vi "usrp TX.vi"() -> ()   [LabVIEW 2019]
uses:
  <instrlib>/niUSRP/niUSRP Write Tx Data (CDB Cluster).vi
  <vilib>/addons/Modulation/Digital/General/MT Generate PSK System Parameters(M).vi
  <vilib>/addons/Modulation/niDMT.lvlib
panel:
  in  "Modulation type":string(combo)="QPSK"
  in  "16-PSK System Parameters 2":T1={"Samples per Symbol"=8, "symbol map"=[], "Differential PSK"=enum."disable", "PSK type"=0} caption="16-PSK System Parameters" {"PSK type" items=["normal", "shifted", "offset"]; "symbol map" format="%.3f"}
  in  "8-PSK System Parameters 2":T1={"Samples per Symbol"=8, "symbol map"=[], "Differential PSK"=enum."disable", "PSK type"=0} caption="8-PSK System Parameters" {"PSK type" items=["normal", "shifted", "offset"]; "symbol map" format="%.3f"}
  in  "QPSK System Parameters 2":T1={"Samples per Symbol"=8, "symbol map"=[], "Differential PSK"=enum."disable", "PSK type"=0} caption="QPSK System Parameters" {"PSK type" items=["normal", "shifted", "offset"]; "symbol map" format="%.3f"}
  in  "BPSK System Parameters 2":T1={"Samples per Symbol"=8, "symbol map"=[], "Differential PSK"=enum."disable", "PSK type"=0} caption="BPSK System Parameters" {"PSK type" items=["normal", "shifted", "offset"]; "symbol map" format="%.3f"}
  in  "PN sequence order\nfor Sync Bits":i32=31 caption="PN sequence order (9)"
  in  "USRP IP address":refnum<k15>="192.168.10.2"
  in  "Packet Pad \n[samples]":i32=200
  out "Number of Packets in Message":i32=46
  in  "Message Text":string="Two roads diverged in a yellow wood,\nAnd sorry I could not travel both\nAnd be one traveler, long I stood\nAnd looked down one as far as I could\nTo where it bent in the undergrowth.\n\nThen took the other, as just as fair,\nAnd having perhaps the better claim,\nBecause it was grassy and wanted wear;\nThough as for that the passing there\nHad worn them really about the same.\n\nAnd both that morning equally lay\nIn leaves no step had trodden black.\nOh, I kept the first for another day!\nYet knowing how way leads on to way,\nI doubted if I should ever come back.\n\nI shall be telling this with a sigh\nSomewhere ages and ages hence:\nTwo roads diverged in a wood, and I--\nI took the one less traveled by,\nAnd that has made all the difference.\n"
  in  "Message Type":bool=TRUE
  in  "Tx Parameters":T2={"Tx IQ Sampling\nRate [s/sec]"=400000.0, "Tx Frequency [Hz]"=915000000.0, "Tx Gain [dB]"=0.0, "Tx Antenna"="TX1"} {"Tx Gain [dB]" format="%#.6p"; "Tx Frequency [Hz]" format="%#.6p"; "Tx IQ Sampling\nRate [s/sec]" format="%#.6p"}
  out "Actual Tx Parameters":T2={"Tx IQ Sampling\nRate [s/sec]"=400000.0, "Tx Frequency [Hz]"=915000000.0, "Tx Gain [dB]"=0.0, "Tx Antenna"="TX1"} {"Tx Gain [dB]" format="%#.6p"; "Tx Frequency [Hz]" format="%#.6p"; "Tx IQ Sampling\nRate [s/sec]" format="%#.6p"}
  in  "Packet Parameters":T3={"Guard Bits "=30, "Sync Bits"=20, "Message Bits"=128}
  out "error out":errorcluster
  out "Constellation Graph":T4(graph)
  in  "autoscale":bool
  out "Transmitted Signal":cluster{"t0":dbl, "dt":dbl, "Y":dbl[]}(graph)
  in  "Queue Length":i32=10
  in  "Blank Frame \n[samples]":i32=500
  in  "Pulse Shaping Filter Parameters":T5={"Alpha"=0.5, "Filter Length"=6, "TX Filter"=enum."Root Raised Cos"} caption="Pulse Shaping Filter" {"Alpha" format="%.2f"}
  out "Symbol Rate [symbols/sec]":dbl=50000.0 format="%#.6p"
  in  "stop":bool
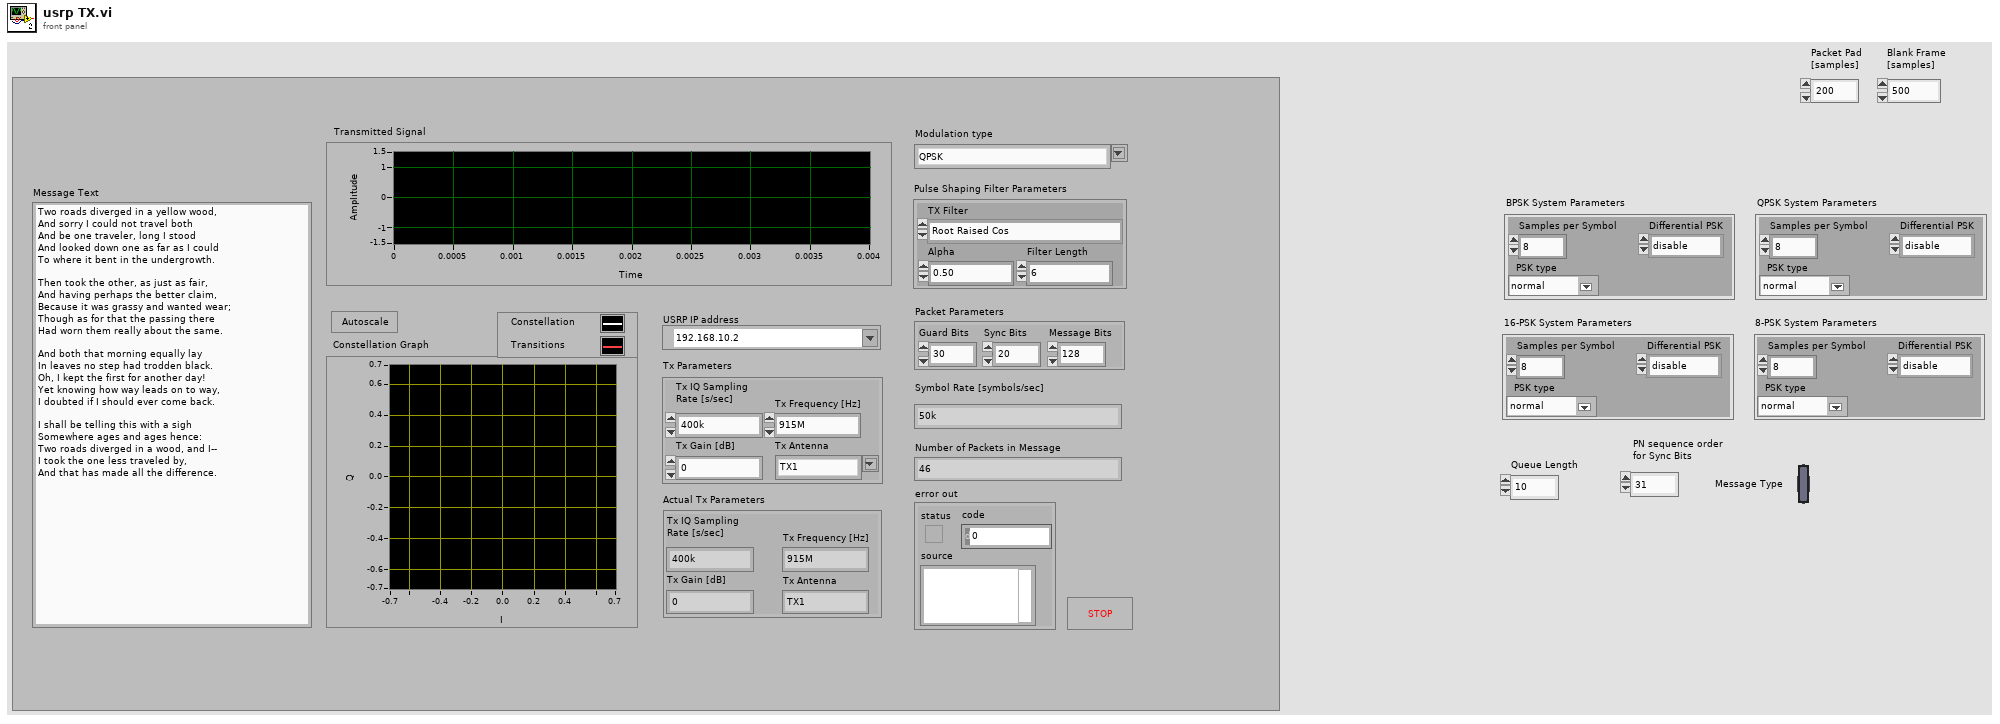
[diagram p1: front panel]
types:
  T1 = cluster{"Samples per Symbol":i32, "symbol map":cdb[], "Differential PSK":enum16{"disable", "enable"}, "PSK type":u16}
  T2 = cluster{"Tx IQ Sampling\nRate [s/sec]":dbl, "Tx Frequency [Hz]":dbl, "Tx Gain [dB]":dbl, "Tx Antenna":string}
  T3 = cluster{"Guard Bits ":i32, "Sync Bits":i32, "Message Bits":i32}
  T4 = cluster{"Decimated Array":dbl[], "Decimated Array":dbl[]}[]
  T5 = cluster{"Alpha":dbl, "Filter Length":i32, "TX Filter":enum16{"none", "Raised Cosine", "Root Raised Cos", "Gaussian"}}
  T6 = cluster{"samples per symbol (16)":i32, "symbol map":cdb[], "differential PSK":enum16{"disable", "enable"}, "PSK type":u16}
  T7 = cluster{"s? t:f":cluster{"t0":dbl, "dt":dbl, "Y":cdb[]}, i32}
  T8 = cluster{"output complex waveform":cluster{"t0":dbl, "dt":dbl, "Y":cdb[]}, i32}
  T9 = cluster{"constellation":dbl[], "oversampled data":dbl[]}[]
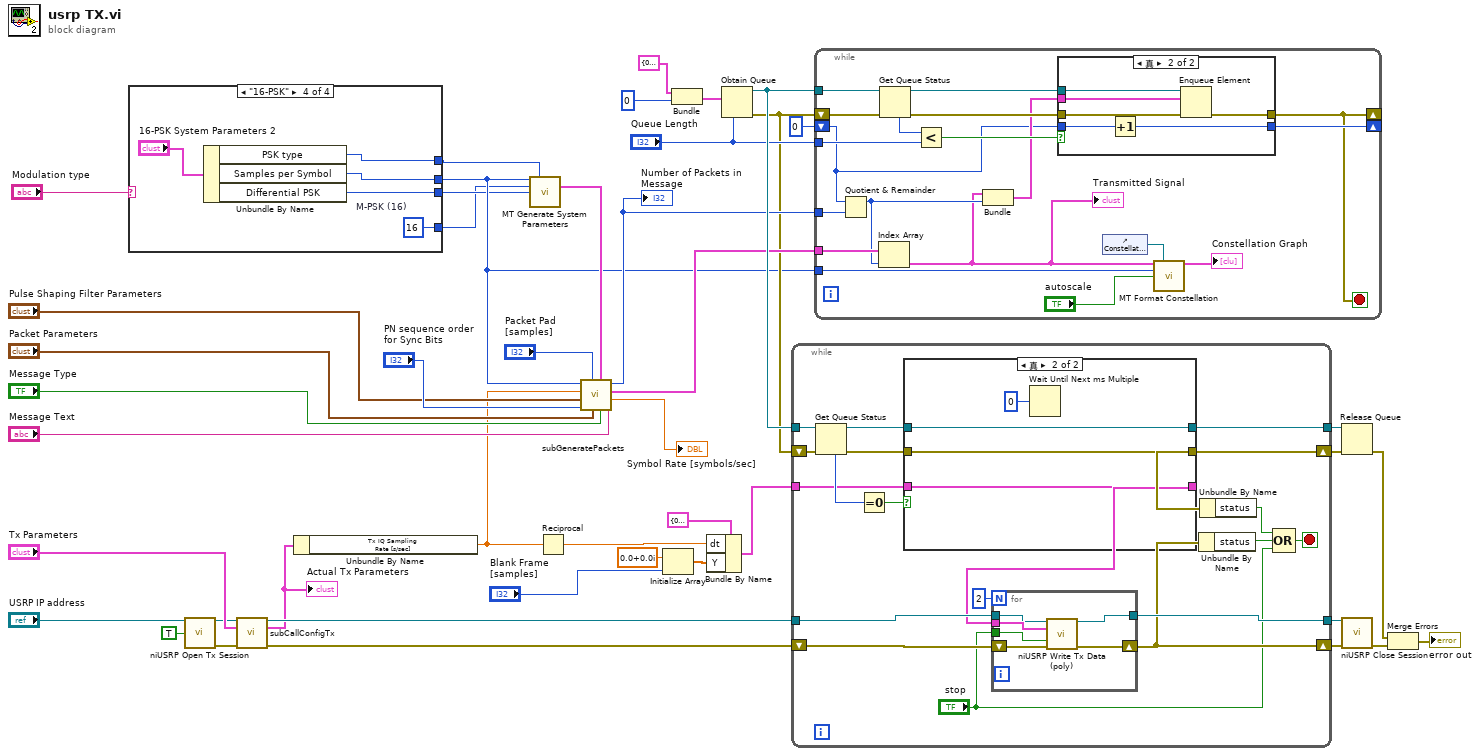
[diagram p0: block diagram]
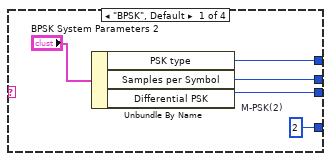
[diagram p2: hidden frame]
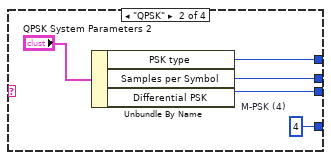
[diagram p3: hidden frame]
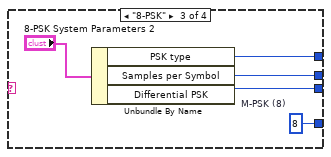
[diagram p4: hidden frame]
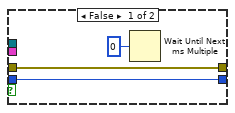
[diagram p5: hidden frame]
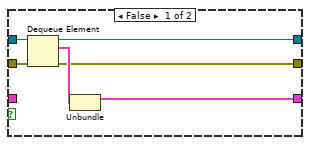
[diagram p6: hidden frame]
diagram:
  n1 = case shown="\"16-PSK\"" "Modulation type" {
    tunnel: [w46 w50 w58 w64] -> w3
    tunnel: [w47 w52 w57 w63] -> w2
    tunnel: [w49 w54 w56 w62] -> w1
    tunnel: [w48 w53 w59 w61] -> w4
    frame "BPSK", Default {
      w49 = 2  # M-PSK(2)
      n2 = Unbundle By Name("BPSK System Parameters 2") -> ("PSK type"=w48:u16, "Samples per Symbol"=w46:i32, "Differential PSK"=w47:enum16{"disable", "enable"})
    }
    frame "QPSK" {
      w54 = 4  # M-PSK (4)
      n3 = Unbundle By Name("QPSK System Parameters 2") -> ("PSK type"=w53:u16, "Samples per Symbol"=w50:i32, "Differential PSK"=w52:enum16{"disable", "enable"})
    }
    frame "8-PSK" {
      w56 = 8  # M-PSK (8)
      n4 = Unbundle By Name("8-PSK System Parameters 2") -> ("PSK type"=w59:u16, "Samples per Symbol"=w58:i32, "Differential PSK"=w57:enum16{"disable", "enable"})
    }
    frame "16-PSK" {
      w62 = 16  # M-PSK (16)
      n5 = Unbundle By Name("16-PSK System Parameters 2") -> ("PSK type"=w61:u16, "Samples per Symbol"=w64:i32, "Differential PSK"=w63:enum16{"disable", "enable"})
    }
  }
  n6 = call <instrlib>:"niUSRP Open Tx Session.vi"("device names"="USRP IP address", "reset"=TRUE) -> ("session handle out"=w18:refnum<k15>, "error out"=w17:errorcluster)  [unwired: 12 in]
  n7 = call "subCallConfigTx.vi"("session handle"=w18, "Tx Parameters"="Tx Parameters", "error in"=w17) -> ("session handle out"=w26:refnum<k15>, "Actual Tx Parameters"=w25:T2, "error out"=w31:errorcluster)  [unwired: 10 in]
  "Actual Tx Parameters" <- w25
  n8 = Unbundle By Name(w25) -> ("Tx IQ Sampling\nRate [s/sec]"=w8:dbl)
  n9 = call-poly <vilib>:"MT Generate System Parameters.vi"("samples per symbol (16)"=w3, "PSK type"=w4, "M-PSK (4)"=w1, "differential PSK"=w2) -> ("PSK system parameters"=w15:T6)  [unwired: 9 in, 2 out]
  n10 = Reciprocal(x=w8) -> (1/x=w27:dbl)
  n11 = call "subGeneratePackets.vi"("Message Text"="Message Text", "Message Type"="Message Type", "PSK system parameters"=w15, "Packet Parameters"="Packet Parameters", "Packet Pad \n[samples]"="Packet Pad \n[samples]", "PN sequence order\nfor Sync Bits"="PN sequence order\nfor Sync Bits", "Pulse Shaping Filter Parameters"="Pulse Shaping Filter Parameters", "Tx IQ Sampling\nRate [s/sec]"=w8, "Samples per Symbol"=w3) -> ("Symbol Rate"=→"Symbol Rate [symbols/sec]":dbl, "Packets"=w33:cluster{"t0":dbl, "dt":dbl, "Y":cdb[]}[], "Number of Packets"=w24:i32)
  "Number of Packets in Message" <- w24
  n12 = Initialize Array(cdb 0.0+0.0i ("element"), "Blank Frame \n[samples]") -> (w41:cdb[])
  n13 = Bundle("s? t:f"=cluster{"t0":dbl, "dt":dbl, "Y":cdb[]} {"t0"=0.0, "dt"=0.0, "Y"=[]}, 0) -> (w36:T7)  [unwired: 1 in]
  n14 = Bundle By Name(cluster=cluster{"t0":dbl, "dt":dbl, "Y":cdb[]} {"t0"=0.0, "dt"=0.0, "Y"=[]} ("s? t:f"), "dt"=w27, "Y"=w41) -> (w40:cluster{"t0":dbl, "dt":dbl, "Y":cdb[]})
  n15 = Obtain Queue(max queue size (-1, unlimited)="Queue Length", element data type=w36) -> (queue out=w42:refnum<queue>, error out=w20:errorcluster)  [unwired: 3 in, 1 out]
  n16 = while {
    tunnel: w26 -> [w74]
    shift-right: [w71] -> w30
    shift-left: w31 -> [w75]
    tunnel: w42 -> [w83]
    tunnel: w40 -> [w80]
    tunnel: [w79] -> w39
    tunnel: [w73] -> w29
    shift-right: [w67] -> w38
    shift-left: w20 -> [w76]
    stop <- w70 stop-if-true
    n17 = Get Queue Status(queue=w83, error in (no error)=w76) -> (queue out=w78:refnum<queue>, error out=w77:errorcluster, # elements in queue=w82:i32)  [unwired: 1 in, 5 out]
    n18 = Equal To 0?(x=w82) -> (x = 0?=w81:bool)
    n19 = case shown="真" w81 {
      tunnel: w80 -> [_ w99]
      tunnel: [w91 w99] -> w65
      tunnel: [w95 w97] -> w79
      tunnel: [w90 w98] -> w67
      tunnel: w78 -> [w94 w97]
      tunnel: w77 -> [w93 w98]
      frame False {
        n20 = Dequeue Element(queue=w94, error in (no error)=w93) -> (queue out=w95:refnum<queue>, element=w92:T7, error out=w90:errorcluster)  [unwired: 1 in, 1 out]
        n21 = Unbundle(w92) -> ("s? t:f"=w91:cluster{"t0":dbl, "dt":dbl, "Y":cdb[]})  [unwired: 1 out]
      }
      frame True {
        n22 = Wait Until Next ms Multiple(millisecond multiple=u32 0) -> ()  [unwired: 1 out]
      }
    }
    n23 = for {
      N: 2 -> [_]
      tunnel: w65 -> [w88]
      tunnel: w74 -> [w87]
      tunnel: [w86] -> w73
      tunnel: "stop" -> [w85]
      shift-right: [w84] -> w71
      shift-left: w75 -> [w89]
      n24 = call-poly <instrlib>:"niUSRP Write Tx Data (poly).vi"("session handle"=w87, "data"=w88, "end of data?"=w85, "error in (no error)"=w89) -> ("session handle out"=w86:refnum<k15>, "error out"=w84:errorcluster)  [unwired: 10 in]
    }
    n25 = Unbundle By Name(w71) -> ("status"=w72:bool)
    n26 = Unbundle By Name(w67) -> ("status"=w66:bool)
    n27 = Compound Arithmetic op=OR(w66, w72, "stop") -> (w70:bool)
  }
  n28 = while {
    tunnel: w42 -> [w118]
    shift-right: [w111] -> _
    shift-left: 0 -> [w107]
    tunnel: w33 -> [w108]
    tunnel: "Queue Length" -> [w110]
    tunnel: w24 -> [w109]
    shift-right: [w105] -> _
    shift-left: w20 -> [w113]
    tunnel: w3 -> [w102]
    stop <- w105 stop-if-true
    n29 = Quotient & Remainder(x=w107, y=w109) -> (x-y*floor(x/y)=w106:i32)  [unwired: 1 out]
    n30 = Index Array "Index Array"(array=w108, index=w106) -> (element=w100:cluster{"t0":dbl, "dt":dbl, "Y":cdb[]})
    "Transmitted Signal" <- w100
    n31 = Get Queue Status(queue=w118, error in (no error)=w113) -> (queue out=w117:refnum<queue>, error out=w114:errorcluster, # elements in queue=w116:i32)  [unwired: 1 in, 5 out]
    n32 = Less?(x=w116, y=w110) -> (x < y?=w115:bool)
    n33 = Bundle("output complex waveform"=w100, w106) -> (w112:T8)  [unwired: 1 in]
    n34 = case shown="真" w115 {
      tunnel: w114 -> [w119 w127]
      tunnel: w117 -> [_ w126]
      tunnel: [w119 w125] -> w105
      tunnel: w112 -> [_ w124]
      tunnel: w107 -> [w121 w123]
      tunnel: [w121 w122] -> w111
      frame False {
        n35 = Wait Until Next ms Multiple(millisecond multiple=u32 0) -> ()  [unwired: 1 out]
      }
      frame True {
        n36 = Increment(x=w123) -> (x+1=w122:i32)
        n37 = Enqueue Element(queue=w126, element=w124, error in (no error)=w127) -> (error out=w125:errorcluster)  [unwired: 1 in, 2 out]
      }
    }
    n38 = control-ref of="Constellation Graph"() -> (w103:refnum<vi>)
    n39 = call <vilib>:"MT Format Constellation.vi"("waveform"=w100, "constellation reference"=w103, "samples per symbol"=w102, "autoscale"="autoscale") -> ("constellation graph"=→"Constellation Graph":T9)  [unwired: 1 in, 10 out]
  }
  n40 = Release Queue(queue=w39, error in (no error)=w38) -> (error out=w14:errorcluster)  [unwired: 3 out]
  n41 = call <instrlib>:"niUSRP Close Session.vi"("session handle"=w29, "error in (no error)"=w30) -> ("error out"=w13:errorcluster)  [unwired: 13 in]
  n42 = Merge Errors(w14, w13) -> (→"error out":errorcluster)
